vi "WPI_ADI_IMU_KalmanFilter.vi"(0 "Data":dbl[](array[numeric]), 5 "dt":dbl format="%#_13g", 7 "Q_Angle":dbl=0.001 format="%#_13g", 9 "Q_Bias":dbl=0.001 format="%#_13g", 11 "R_Measure":dbl=0.01 format="%#_13g", 12 "Restrict? (f)":bool) -> (4 "Roll":dbl, 6 "Pitch":dbl)   [LabVIEW 2015]
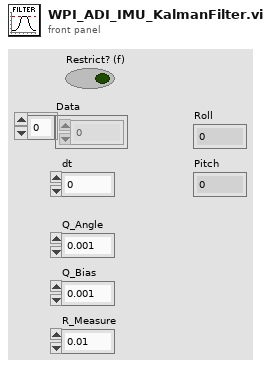
[diagram p1: front panel]
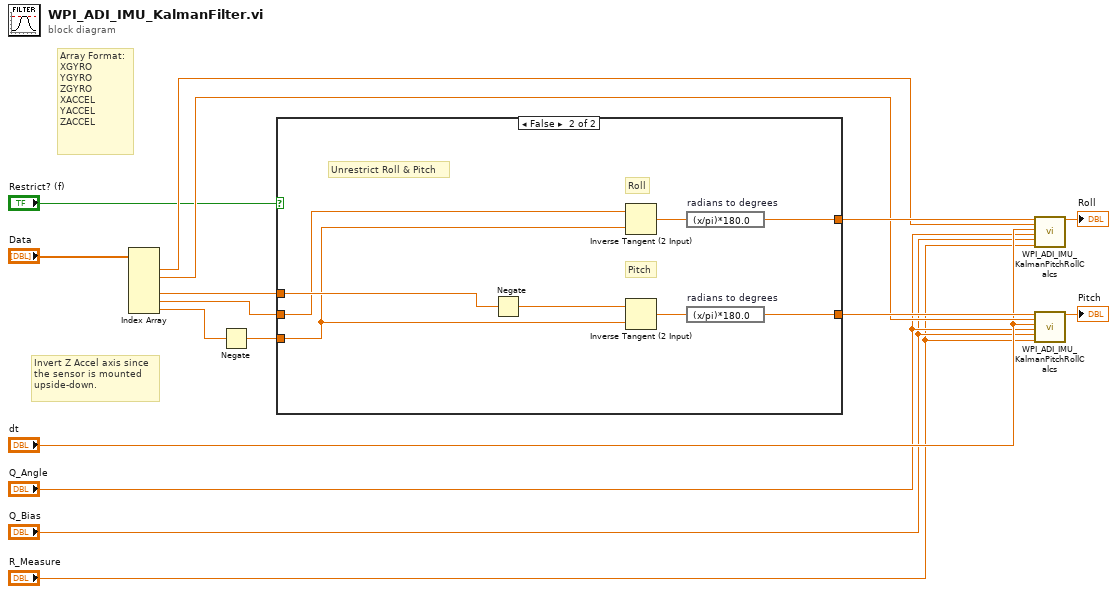
[diagram p0: block diagram]
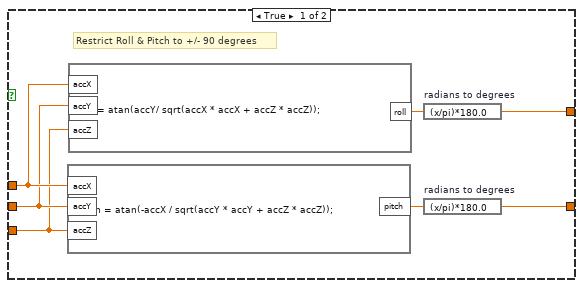
[diagram p2: hidden frame]
diagram:
  # "Array Format:\nXGYRO\nYGYRO\nZGYRO\nXACCEL\nYACCEL\nZACCEL"
  # "Invert Z Accel axis since\nthe sensor is mounted \nupside-down."
  n1 = Index Array(array="Data") -> (element #1=w11:dbl, element #2=w10:dbl, element #4=w15:dbl, element #5=w14:dbl, element #6=w4:dbl)  [unwired: 6 in, 1 out]
  n2 = Negate(x=w4) -> (-x=w5:dbl)
  n3 = case shown="False" "Restrict? (f)" {
    tunnel: w15 -> [w21 w30]
    tunnel: w14 -> [w20 w26]
    tunnel: w5 -> [w19 w25]
    tunnel: [w18 w28] -> w13
    tunnel: [w17 w27] -> w12
    frame True {
      # "Restrict Roll & Pitch to +/- 90 degrees"
      n4 = formula code="pitch = atan(-accX / sqrt(accY * accY + accZ * accZ));"("accX"=w21, "accY"=w20, "accZ"=w19) -> ("pitch"=w23:dbl)
      n5 = formula code="roll = atan(accY/ sqrt(accX * accX + accZ * accZ));"("accX"=w21, "accY"=w20, "accZ"=w19) -> ("roll"=w22:dbl)
      n6 = expression code="(x/pi)*180.0" "radians to degrees"(w22) -> (w18:dbl)
      n7 = expression code="(x/pi)*180.0" "radians to degrees"(w23) -> (w17:dbl)
    }
    frame False {
      # "Unrestrict Roll & Pitch"
      # "Pitch"
      # "Roll"
      n8 = Negate(x=w30) -> (-x=w24:dbl)
      n9 = Inverse Tangent (2 Input)(1:w25, 2:w26) -> (0:w31:dbl)
      n10 = Inverse Tangent (2 Input)(1:w25, 2:w24) -> (0:w29:dbl)
      n11 = expression code="(x/pi)*180.0" "radians to degrees"(w31) -> (w28:dbl)
      n12 = expression code="(x/pi)*180.0" "radians to degrees"(w29) -> (w27:dbl)
    }
  }
  n13 = call "WPI_ADI_IMU_KalmanPitchRollCalcs.vi"("Accel"=w13, "Gyro"=w11, "dt (ms)"="dt", "Q_Angle"="Q_Angle", "Q_Bias"="Q_Bias", "R_Measure"="R_Measure") -> ("Filtered"=→"Roll":dbl)  [unwired: 13 in]
  n14 = call "WPI_ADI_IMU_KalmanPitchRollCalcs.vi"("Accel"=w12, "Gyro"=w10, "dt (ms)"="dt", "Q_Angle"="Q_Angle", "Q_Bias"="Q_Bias", "R_Measure"="R_Measure") -> ("Filtered"=→"Pitch":dbl)  [unwired: 13 in]
